vi "Multiple_TIFFBlock.vi"() -> ()   [LabVIEW 2011]
panel:
  out "Numeric":i32
  in  "Array":T1(array[cluster])
  in  "Output file":u16(ring)=1 items=["Big-Endian"=0, "Native"=1, "Little-Endian"=2, "BigTiff-Big-Endian"=256, "Bigtiff,Native"=257, "Biftiff,Littleendian"=258]
  in  "offset":dbl=3200.0
  in  "Blocksize":i16=8
  # "Max-Min>Threshold"
  # "eher weniger, schlechterer Contrast1000"
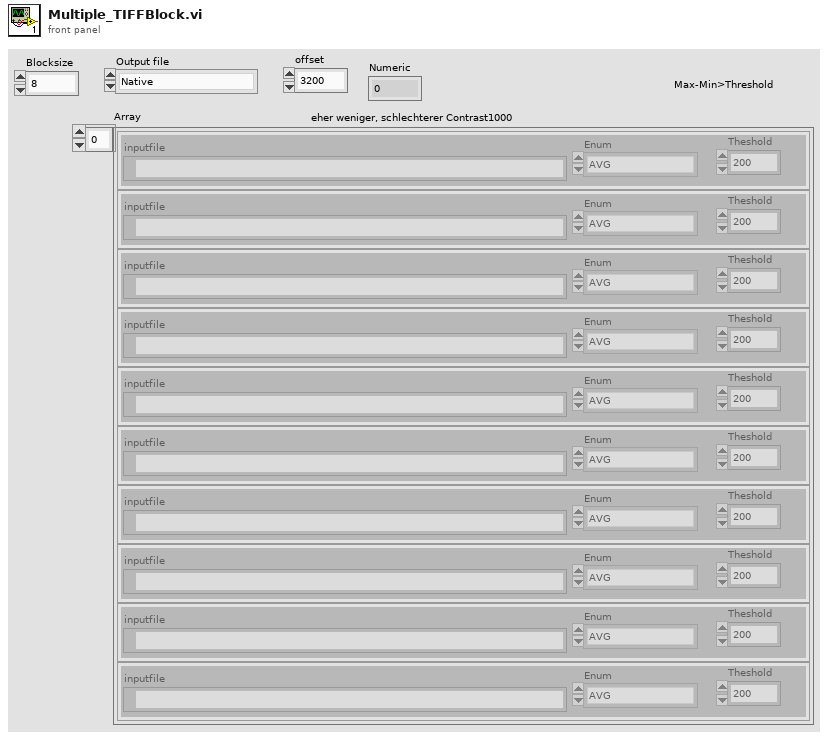
[diagram p1: front panel]
types:
  T1 = cluster{"inputfile":path, "Enum":enum16{"AVG", "STD", "Contrast1000"}, "Theshold":dbl}[]
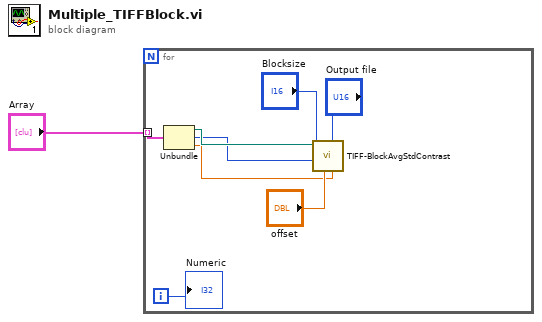
[diagram p0: block diagram]
diagram:
  n1 = for {
    tunnel: "Array" -> [w6] mode=indexing
    i -> [w2]
    n2 = Unbundle(w6) -> ("inputfile"=w5:path, "Enum"=w4:enum16{"AVG", "STD", "Contrast1000"}, "Theshold"=w3:dbl)
    n3 = call "TIFF-BlockAvgStdContrast.vi"("Theshold"=w3, "Output file"="Output file", "offset"="offset", "Enum"=w4, "Blocksize"="Blocksize", "inputfile"=w5) -> ()  [unwired: 4 in, 1 out]
    "Numeric" <- w2
  }
